vi "Destroy User Events.vi"(11 "VG-VNA_GUI in":refnum<class "VG-VNA_GUI.lvclass">) -> (3 "VG-VNA_GUI out":refnum<class "VG-VNA_GUI.lvclass">)   [LabVIEW 2020, in "VG-VNA_GUI.lvlib" / "VG-VNA_GUI.lvclass"]
uses:
  VG-VNA_GUI.lvclass
  VG-VNA_GUI.lvclass/VG-VNA_GUI.ctl
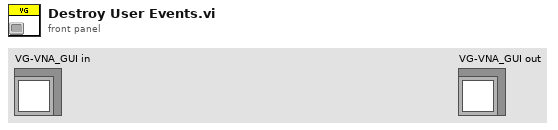
[diagram p1: front panel]
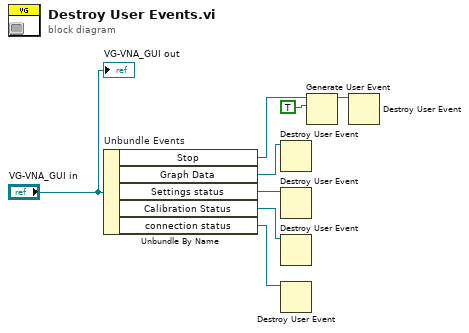
[diagram p0: block diagram]
diagram:
  n1 = Unbundle By Name "Unbundle Events"("VG-VNA_GUI in") -> ("Stop"=w6:refnum<user-event>, "Graph Data"=w5:refnum<user-event>, "Settings status"=w3:refnum<user-event>, "Calibration Status"=w2:refnum<user-event>, "connection status"=w1:refnum<user-event>)
  n2 = Destroy User Event(user event=w5) -> ()  [unwired: 1 in, 1 out]
  n3 = Destroy User Event(user event=w3) -> ()  [unwired: 1 in, 1 out]
  n4 = Destroy User Event(user event=w2) -> ()  [unwired: 1 in, 1 out]
  n5 = Destroy User Event(user event=w1) -> ()  [unwired: 1 in, 1 out]
  n6 = Generate User Event(user event=w6, event data cluster=TRUE ("event data")) -> (user event out=w7:refnum<user-event>)  [unwired: 2 in, 1 out]
  n7 = Destroy User Event(user event=w7) -> ()  [unwired: 1 in, 1 out]
  "VG-VNA_GUI out" <- "VG-VNA_GUI in"
